vi "加标模块单控对话框.vi"(10 "数组":refnum<vi>[](array[refnum]), 11 "标题":string="加标模块") -> ()   [LabVIEW 2016, in "质控单元.lvlib"]
panel:
  in  "慢速到液位":bool
  in  "排液":bool
  in  "退出":bool
  in  "柱塞泵":bool
  in  "排液":bool
  in  "搅拌":bool
  in  "进样调速":bool
  in  "进样":bool
  in  "停止":bool
  in  "加标启动":bool
  # "手动控制"
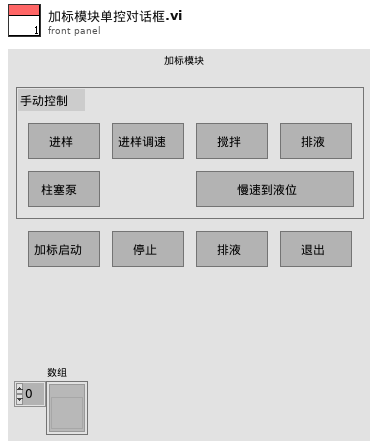
[diagram p1: front panel]
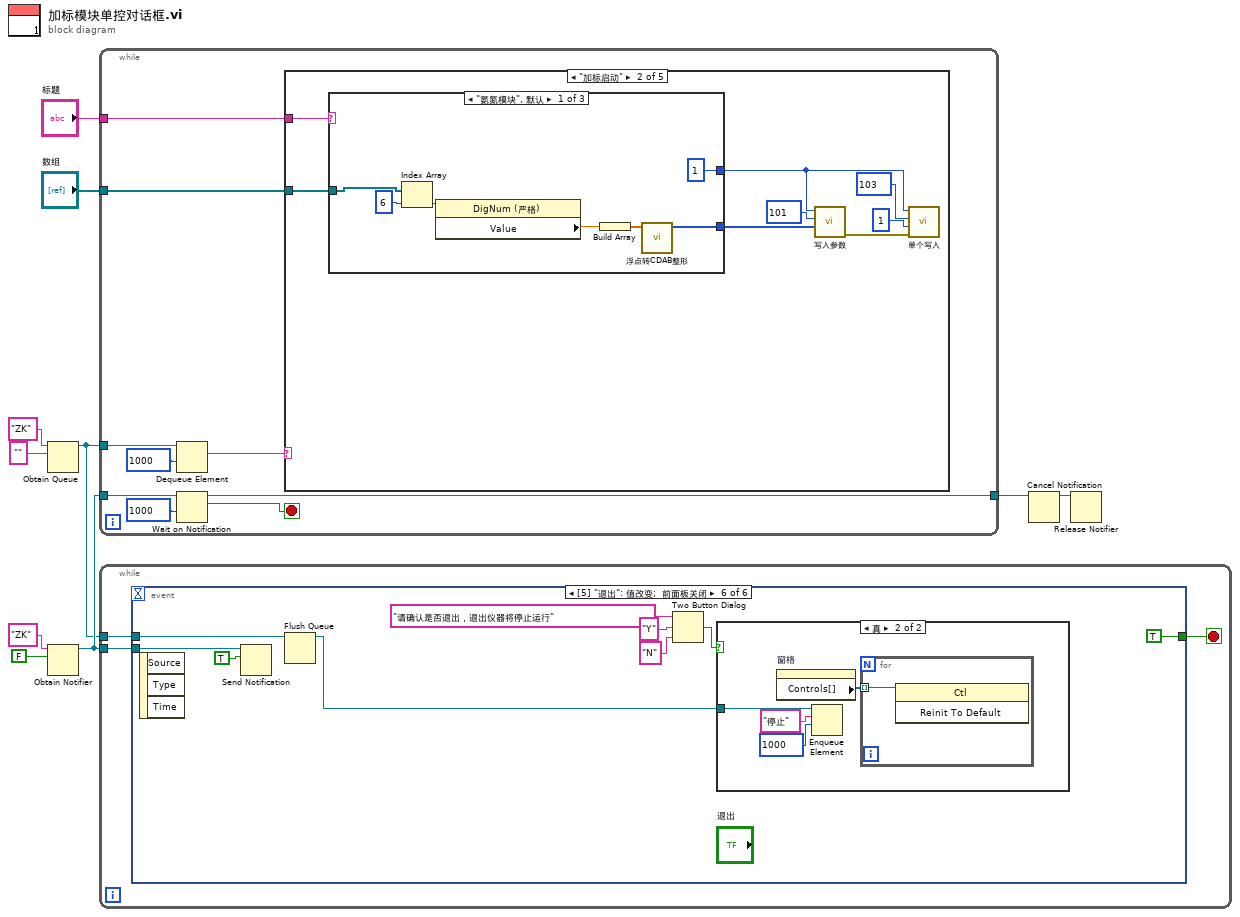
[diagram p0: block diagram]
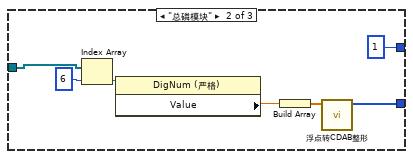
[diagram p3: hidden frame]
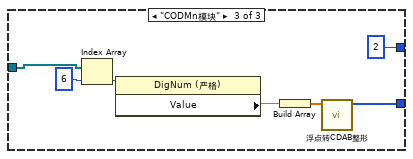
[diagram p4: hidden frame]
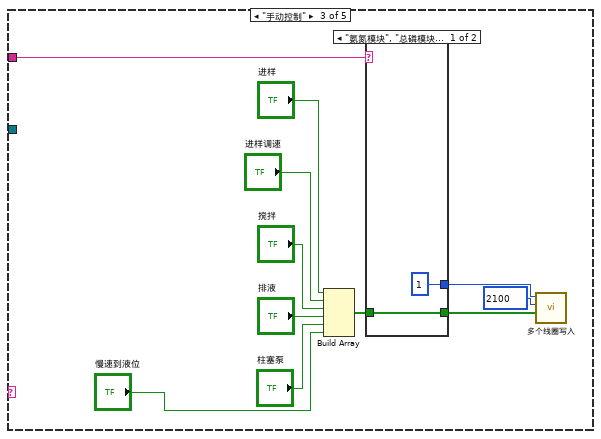
[diagram p5: hidden frame]
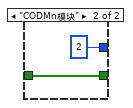
[diagram p6: hidden frame]
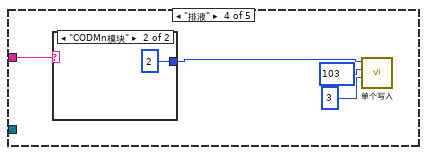
[diagram p7: hidden frame]
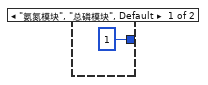
[diagram p8: hidden frame]
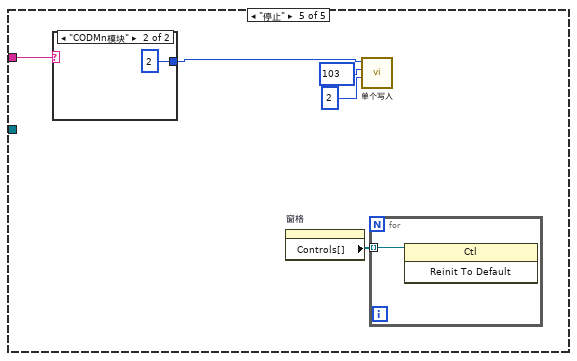
[diagram p9: hidden frame]
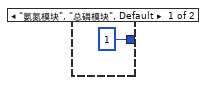
[diagram p10: hidden frame]
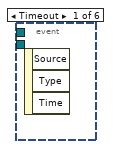
[diagram p11: hidden frame]
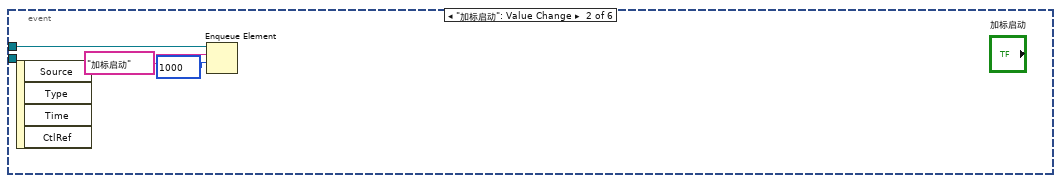
[diagram p12: hidden frame]
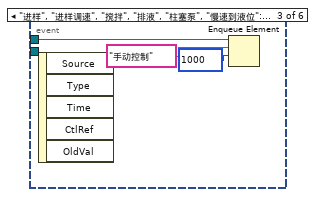
[diagram p13: hidden frame]
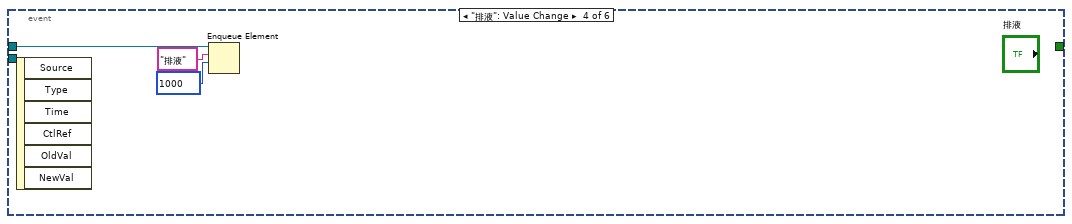
[diagram p14: hidden frame]
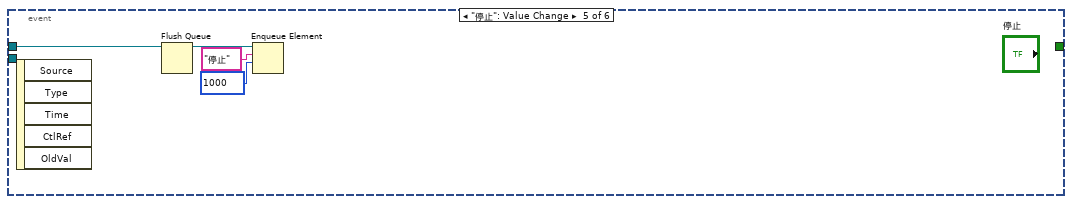
[diagram p15: hidden frame]
diagram:
  n1 = Obtain Queue(name (unnamed)="ZK" ("名称（未命名）"), element data type="" ("名称（未命名）")) -> (queue out=w3:refnum<queue>)  [unwired: 3 in, 2 out]
  n2 = Obtain Notifier(name (unnamed)="ZK" ("名称（未命名）"), notification data type=FALSE) -> (notifier out=w8:refnum<notifier>)  [unwired: 2 in, 2 out]
  n3 = while {
    tunnel: w8 -> [w19]
    tunnel: [w17] -> w7
    tunnel: w3 -> [w16]
    tunnel: "数组" -> [w11]
    tunnel: "标题" -> [w12]
    stop <- w18 stop-if-true
    n4 = Dequeue Element(queue=w16, timeout in ms (-1)=1000 ("超时毫秒(-1)")) -> (element=w15:string)  [unwired: 1 in, 3 out]
    n5 = Wait on Notification(notifier=w19, timeout in ms (-1)=1000 ("超时毫秒(-1)")) -> (notifier out=w17:refnum<notifier>, notification=w18:bool)  [unwired: 2 in, 2 out]
    n6 = case shown="\"加标启动\"" w15 {
      tunnel: w12 -> [_ w21 w49 w64 w71]
      tunnel: w11 -> [_ w20 _ _ _]
      frame Default {
      }
      frame "加标启动" {
        n7 = case shown="\"氨氮模块\", 默认" w21 {
          tunnel: w20 -> [w30 w37 w44]
          tunnel: [w29 w36 w43] -> w23
          tunnel: [u8 1 ("Slave ID") u8 1 ("Slave ID") u8 2 ("Slave ID")] -> w27
          frame "氨氮模块", Default {
            n8 = Index Array(array=w30, index=6 ("索引")) -> (element=w34:refnum<vi>)
            n9 = property class="DigNum (严格)"(reference=w34) -> ("Value"=w33:dbl)  [unwired: 1 in, 2 out]
            n10 = Build Array(w33) -> (w32:dbl[])
            n11 = call "浮点转CDAB整形.vi"("浮点数"=w32) -> ("CDAB整形输出"=w29:u16[])  [unwired: 10 in]
          }
          frame "总磷模块" {
            n12 = Index Array(array=w37, index=6 ("索引")) -> (element=w41:refnum<vi>)
            n13 = property class="DigNum (严格)"(reference=w41) -> ("Value"=w40:dbl)  [unwired: 1 in, 2 out]
            n14 = Build Array(w40) -> (w39:dbl[])
            n15 = call "浮点转CDAB整形.vi"("浮点数"=w39) -> ("CDAB整形输出"=w36:u16[])  [unwired: 10 in]
          }
          frame "CODMn模块" {
            n16 = Index Array(array=w44, index=6 ("索引")) -> (element=w48:refnum<vi>)
            n17 = property class="DigNum (严格)"(reference=w48) -> ("Value"=w47:dbl)  [unwired: 1 in, 2 out]
            n18 = Build Array(w47) -> (w46:dbl[])
            n19 = call "浮点转CDAB整形.vi"("浮点数"=w46) -> ("CDAB整形输出"=w43:u16[])  [unwired: 10 in]
          }
        }
        n20 = call "写入参数.vi"("values"=w23, "starting address"=u16 101, "Slave ID"=w27) -> ("error out"=w22:errorcluster)  [unwired: 8 in]
        n21 = call "单个写入.vi"("Error in"=w22, "value"=u16 1, "address"=u16 103, "Slave ID"=w27) -> ()  [unwired: 7 in, 1 out]
      }
      frame "手动控制" {
        n22 = Build Array("进样", "进样调速", "搅拌", "排液", "柱塞泵", "慢速到液位") -> (w55:bool[])
        n23 = case shown="\"氨氮模块\", \"总磷模块\", 默认" w49 {
          tunnel: w55 -> [w61 w63]
          tunnel: [w61 w63] -> w56
          tunnel: [u8 1 ("Slave ID") u8 2 ("Slave ID")] -> w58
          frame "氨氮模块", "总磷模块", Default {
          }
          frame "CODMn模块" {
          }
        }
        n24 = call "多个线圈写入.vi"("values"=w56, "starting address"=u16 2100, "Slave ID"=w58) -> ()  [unwired: 8 in, 1 out]
      }
      frame "排液" {
        n25 = case shown="\"CODMn模块\"" w64 {
          tunnel: [u8 1 ("Slave ID") u8 2 ("Slave ID")] -> w65
          frame "氨氮模块", "总磷模块", Default {
          }
          frame "CODMn模块" {
          }
        }
        n26 = call "单个写入.vi"("value"=u16 3, "address"=u16 103, "Slave ID"=w65) -> ()  [unwired: 8 in, 1 out]
      }
      frame "停止" {
        n27 = case shown="\"CODMn模块\"" w71 {
          tunnel: [u8 1 ("Slave ID") u8 2 ("Slave ID")] -> w72
          frame "氨氮模块", "总磷模块", Default {
          }
          frame "CODMn模块" {
          }
        }
        n28 = property on="窗格" class="Pane"() -> ("Controls[]"=w70:refnum<vi>[])  [unwired: 2 in, 2 out]
        n29 = call "单个写入.vi"("value"=u16 2, "address"=u16 103, "Slave ID"=w72) -> ()  [unwired: 8 in, 1 out]
        n30 = for {
          tunnel: w70 -> [w75] mode=indexing
          n31 = invoke class="Ctl" method="Reinit To Default"(reference=w75) -> ()  [unwired: 2 in, 3 out]
        }
      }
    }
  }
  n32 = while {
    tunnel: w8 -> [w79]
    tunnel: w3 -> [w78]
    stop <- w80 stop-if-true
    n33 = event shown="[5] \"退出\": 值改变;  前面板关闭" {
      selector: _ -> [_ _ _ _ _ _]
      dyn-events: _ -> [_ _ _ _ _ _]
      timeout: _ -> [_ _ _ _ _ _]
      tunnel: [_ _ _ _ _ TRUE] -> w80
      tunnel: w79 -> [_ _ _ _ _ w96]
      tunnel: w78 -> [_ w83 w84 w87 w92 w95]
      event Timeout {
        n34 = event-data() -> ()  [unwired: 1 in, 3 out]
      }
      event "加标启动": Value Change {
        n35 = event-data() -> ()  [unwired: 1 in, 4 out]
        n36 = Enqueue Element(queue=w83, element="加标启动" ("元素"), timeout in ms (-1)=1000 ("超时毫秒(-1)")) -> ()  [unwired: 1 in, 3 out]
      }
      event "进样", "进样调速", "搅拌", "排液", "柱塞泵", "慢速到液位": Value Change {
        n37 = event-data() -> ()  [unwired: 1 in, 5 out]
        n38 = Enqueue Element(queue=w84, element="手动控制" ("元素"), timeout in ms (-1)=1000 ("超时毫秒(-1)")) -> ()  [unwired: 1 in, 3 out]
      }
      event "排液": Value Change {
        n39 = event-data() -> ()  [unwired: 1 in, 6 out]
        n40 = Enqueue Element(queue=w87, element="排液" ("元素"), timeout in ms (-1)=1000 ("超时毫秒(-1)")) -> ()  [unwired: 1 in, 3 out]
      }
      event "停止": Value Change {
        n41 = event-data() -> ()  [unwired: 1 in, 5 out]
        n42 = Flush Queue(queue=w92) -> (queue out=w91:refnum<queue>)  [unwired: 1 in, 2 out]
        n43 = Enqueue Element(queue=w91, element="停止" ("元素"), timeout in ms (-1)=1000 ("超时毫秒(-1)")) -> ()  [unwired: 1 in, 3 out]
      }
      event "退出": Value Change; Panel Close {
        n44 = event-data() -> ()  [unwired: 1 in, 3 out]
        n45 = Send Notification(notification=TRUE ("通知"), notifier=w96) -> ()  [unwired: 1 in, 2 out]
        n46 = Flush Queue(queue=w95) -> (queue out=w94:refnum<queue>)  [unwired: 1 in, 2 out]
        n47 = Two Button Dialog(message="请确认是否退出，退出仪器将停止运行" ("消息"), 1:"N" ("F按钮名称（“取消”）"), 2:"Y" ("T按钮名称（“确定”）")) -> (T button?=w98:bool)
        n48 = case shown="真" w98 {
          tunnel: w94 -> [_ w103]
          frame False {
          }
          frame True {
            n49 = property on="窗格" class="Pane"() -> ("Controls[]"=w106:refnum<vi>[])  [unwired: 2 in, 2 out]
            n50 = Enqueue Element(queue=w103, element="停止" ("元素"), timeout in ms (-1)=1000 ("超时毫秒(-1)")) -> ()  [unwired: 1 in, 3 out]
            n51 = for {
              tunnel: w106 -> [w107] mode=indexing
              n52 = invoke class="Ctl" method="Reinit To Default"(reference=w107) -> ()  [unwired: 2 in, 3 out]
            }
          }
        }
      }
    }
  }
  n53 = Cancel Notification(0:w7) -> (8:w6:refnum<notifier>)  [unwired: 1 in, 2 out]
  n54 = Release Notifier(notifier=w6) -> ()  [unwired: 2 in, 3 out]
